vi "Chamber controller Dec 8 2016.vi"() -> ()   [LabVIEW 2014]
uses:
  <vilib>/Instr/_visa.llb/VISA Configure Serial Port (Instr).vi
  Environmental Chamber LabVIEW and Instruments/Drivers and Software/Keithley 2100 Series/Public/Configure/Configure 2 Wire Resistance.vi
  <vilib>/Utility/file.llb/Write To Spreadsheet File (string).vi
  <vilib>/Utility/file.llb/Read From Spreadsheet File (string).vi
  Environmental Chamber LabVIEW and Instruments/Drivers and Software/keithley_6430/Keithley 6430/Public/Data/Read (Single Point).vi
  Environmental Chamber LabVIEW and Instruments/Drivers and Software/LabVIEW 8.2 Drivers/keithley_24xx/Keithley 24XX/Public/Data/Read (Single Point).vi
  Environmental Chamber LabVIEW and Instruments/Drivers and Software/keithley_24xx/Keithley 24XX/Keithley 24XX.lvlib
  Environmental Chamber LabVIEW and Instruments/Drivers and Software/keithley_6430/Keithley 6430/Keithley 6430.lvlib
  Environmental Chamber LabVIEW and Instruments/Drivers and Software/Keithley 2100 Series/Keithley 2100 Series.lvlib
panel:
  out "pressure chart":cluster{"pressure":dbl}(graph)
  out "arduino qcm stack plot":T1(graph)
  in  "K-2420 tab control":enum32{"K-2420 Measure", "K-2420 Apply bias"}(tab)
  out "K-2420 2":cluster{"Resistance":sgl}(graph)
  in  "Applied Voltage (V)":dbl min=-5.0 max=5.0 step=5e-06
  out "K-2420 4":cluster{"Applied Voltage (V)":dbl}(graph)
  out "saving data?":bool
  in  "Data logging settings":T2={"Save during sequence only"=TRUE, "Save now"=FALSE, "sec between data points"=0.0, "Current data file path"=path "", "Save sample names"={"QCM1"="", "QCM2"="", "QCM3"="", "QCM4"="", "QCM5"="", "QCM6"="", "SRS"="", "K-2420"="", "K-6430"="", "K-2100"=""}, "Experiment Notes"="", "Cluster"={"Gas:"="CO2", "Vapor:"="H2O"}} {"sec between data points" min=0.0 max=30.0 format="%#_13g"}
  in  "Sequence cluster":T3={"Save sequence"=FALSE, "Clear sequence"=FALSE, "Import sequence file"=FALSE, "Tare elapsed time"=TRUE, "Run Sequence"=FALSE, "Stop program when sequence ends"=TRUE, "User-defined\nsequence"=[], "Sequence end time"="", "Sequence\npreview"=[], "Current\nstep"=0, "Display"=0} caption="Sequence settings" {"Display" items=["pressure", "gas flow", "vapor flow", "bias"]}
  in  "Pressure parameters cluster":T4={"valve % open"=100.0, "Desired pressure"=0.0, "Vapor sccm"=0.0, "Gas sccm"=0.0, "Valve mode"=enum."% Open", "Pressure Mode"=enum."Abs. pressure", "analyte partial pressure"=23.8, "Turbo pump\nauto on"=TRUE, "Valve position (%)"=0.0, "read pressure"=0.0, "read vapor flow"=0.0, "read gas flow"=0.0} caption="Pressure settings" {"read gas flow" format="%#_3g"; "read vapor flow" format="%#_3g"; "read pressure" format="%#_7f"; "Valve position (%)" format="%#_3g"; "analyte partial pressure" min=0.0 max=100.0 step=5.0; "Gas sccm" min=0 max=200 step=5; "Vapor sccm" min=0 max=200 step=5; "Desired pressure" min=0.0 max=760.0 step=5.0; "valve % open" min=0.0 max=100.0 step=5.0 format="%#_2f"}
  out "J-KEM temp chart":dbl(graph)
  out "Elapsed time (min)":dbl
  out "State date/time":string caption="Start time"
  out "K-2100 (Ohm)":cluster{"Measurement":dbl}(graph) caption="K-2100"
  out "K-6430":cluster{"Measurement":dbl}(graph)
  in  "Gate time (s)":enum16{"0.1", "1.0 ", "10"}(ring)=enum."1.0 "
  out "Hz":dbl format="%#.7f"
  out "QCM plot":T5(graph)
  in  "Stop":bool
  in  "Clear all charts":bool
  out "ArduinoQCM cluster":T6 caption="Arduino QCM" {"6" format="%_8g"; "5" format="%_8g"; "4" format="%_8g"; "3" format="%_8g"; "2" format="%_8g"; "1" format="%#_10g"}
  out "O2 sensor output":dbl[](array[numeric]) caption="atm\nTorr"
  in  "rapidox O2 Sensor":bool
  in  "setnag O2 Pump":bool
  in  "Baud Rate 2":i32(ring)=2 items=["2400", "4800", "9600", "19200", "38400", "57600", "115200"]
  in  "Com Port":i32(ring) items=["Com 1", "Com 2", "Com 3", "Com 4", "Com 5", "Com 6", "COM 7", "COM 8", "COM 9", "COM 10", "COM 11", "COM 12", "com 13", "COM 14"]
  in  "Com Port 2":i32(ring) items=["Com 1", "Com 2", "Com 3", "Com 4", "Com 5", "Com 6", "COM 7", "COM 8", "COM 9", "COM 10", "COM 11", "COM 12", "com 13", "COM 14"]
  out "Waveform Chart":cluster{dbl}(graph)
  out "O2 Concentration (PPM)":dbl
  out "Waveform Chart 6":cluster{dbl}(graph)
  # "Currently Unused"
  # "SRS"
  # "100%"
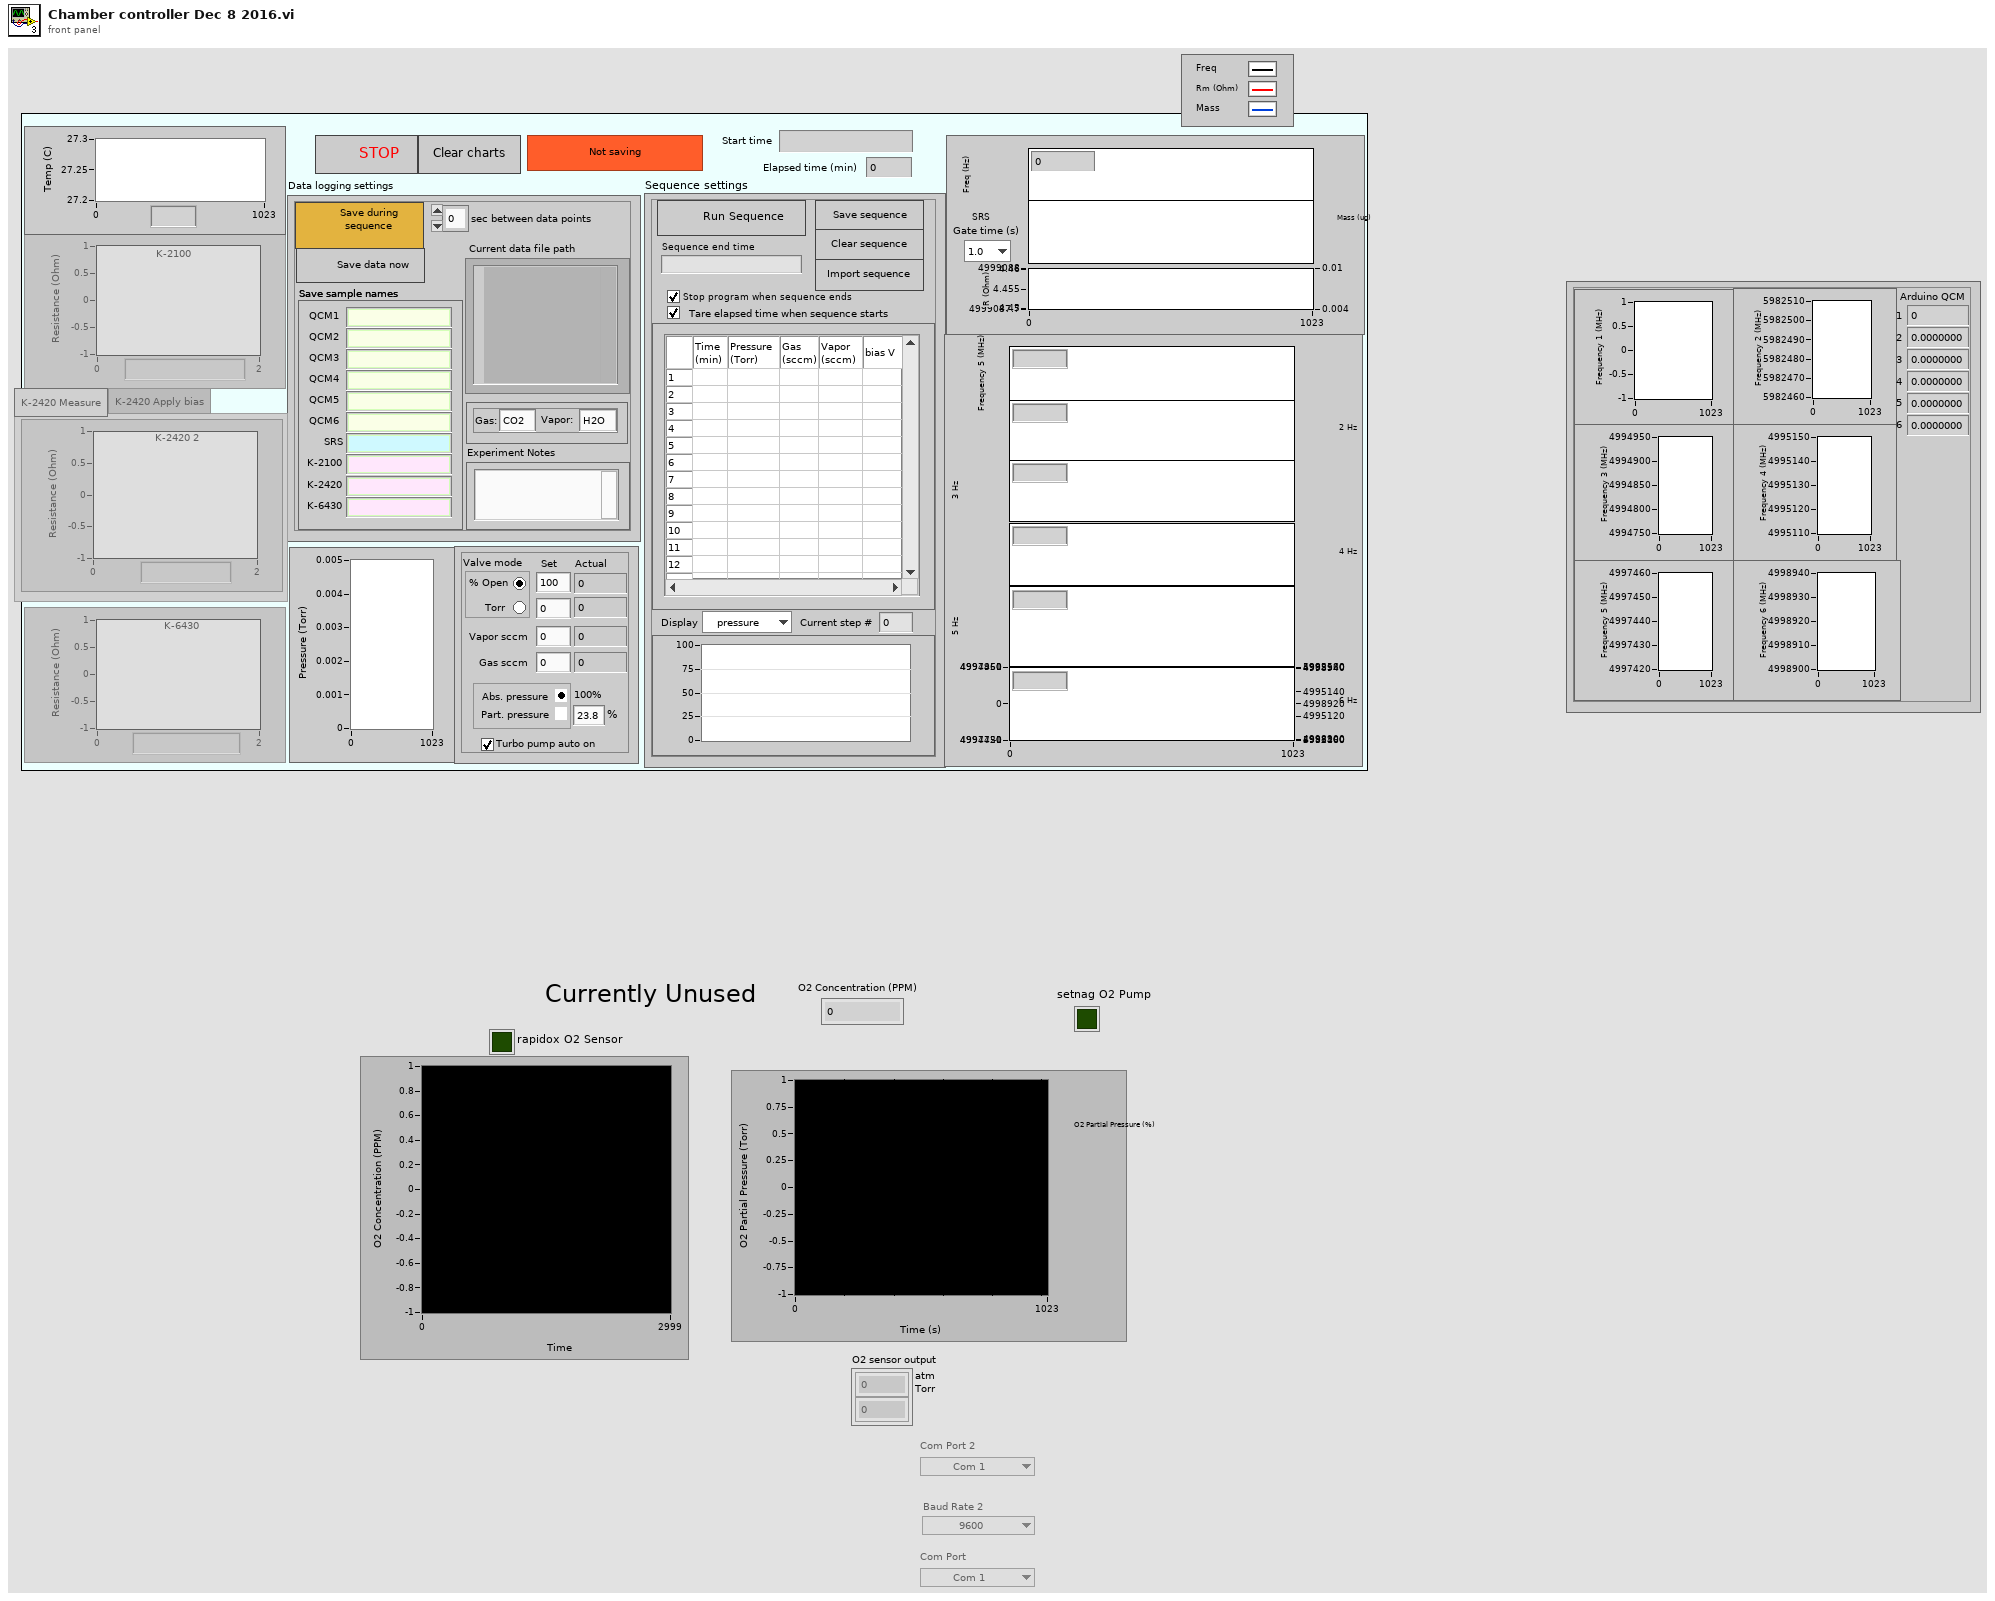
[diagram p1: front panel]
types:
  T1 = cluster{"mean":dbl, "mean":dbl, "mean":dbl, "mean":dbl, "mean":dbl, "mean":dbl}
  T2 = cluster{"Save during sequence only":bool, "Save now":bool, "sec between data points":dbl, "Current data file path":path, "Save sample names":cluster{"QCM1":string, "QCM2":string, "QCM3":string, "QCM4":string, "QCM5":string, "QCM6":string, "SRS":string, "K-2420":string, "K-6430":string, "K-2100":string}, "Experiment Notes":string, "Cluster":cluster{"Gas:":string, "Vapor:":string}}
  T3 = cluster{"Save sequence":bool, "Clear sequence":bool, "Import sequence file":bool, "Tare elapsed time":bool, "Run Sequence":bool, "Stop program when sequence ends":bool, "User-defined\nsequence":string[][], "Sequence end time":string, "Sequence\npreview":cluster{dbl[], dbl[]}[], "Current\nstep":i32, "Display":u16}
  T4 = cluster{"valve % open":dbl, "Desired pressure":dbl, "Vapor sccm":sgl, "Gas sccm":sgl, "Valve mode":enum32{"% Open", "Torr "}, "Pressure Mode":enum32{"Abs. pressure", " Part. pressure"}, "analyte partial pressure":dbl, "Turbo pump\nauto on":bool, "Valve position (%)":dbl, "read pressure":dbl, "read vapor flow":dbl, "read gas flow":dbl}
  T5 = cluster{"Frequency out":dbl, "Numeric Control":dbl, "Resistance out":dbl}
  T6 = cluster{"arduino qcm 1":dbl, "1":dbl, "arduino qcm 2":dbl, "2":dbl, "arduino qcm 3":dbl, "3":dbl, "arduino qcm 4":dbl, "4":dbl, "arduino qcm 5":dbl, "5":dbl, "arduino qcm 6":dbl, "6":dbl}
  T7 = cluster{"Keithley 6430":bool, "J-KEM":bool, "Keithley 2420":bool, "Keithley 2100":bool, "SRS QCM":bool, "Pressure control":bool, "Arduino":bool}
  T8 = cluster{"Arduino 1":refnum<visa-resource-name>, "Arduino 2":refnum<visa-resource-name>, "Arduino 3":refnum<visa-resource-name>, "Arduino 4":refnum<visa-resource-name>, "Arduino 5":refnum<visa-resource-name>, "Arduino 6":refnum<visa-resource-name>}
  T9 = enum8{"Enabled", "Disabled", "Disabled and Grayed Out"}
  T10 = enum16{"open", "open or create", "create or replace", "create", "open (read only)"}
  T11 = enum16{"no parity", "odd parity", "even parity", "mark parity", "space parity"}
  T12 = cluster{"mean":dbl, "mean":dbl, "mean":dbl, "mean":dbl, "mean":dbl, "mean":dbl}[]
  T13 = cluster{"Frequency out":dbl, "Numeric Control":dbl, "Resistance out":dbl}[]
  T14 = cluster{"String":string, "String":string, "String":string}
  T15 = cluster{bool, "task out":refnum<k21>, "error out":errorcluster, "task out":refnum<k21>, "error out":errorcluster, "turbo pump":refnum<visa-resource-name>, "error out":errorcluster}
  T16 = cluster{bool, "task out":refnum<k21>, "error out":errorcluster, "task out":refnum<k21>, "error out":errorcluster, "VISA resource name out":refnum<visa-resource-name>, "error out":errorcluster}
  T17 = cluster{bool, "VISA resource name":refnum<visa-resource-name>, "error out":errorcluster}
  T18 = cluster{bool, "VISA resource name out":refnum<visa-resource-name>, "error out":errorcluster}
  T19 = cluster{"VISA resource name out":refnum<visa-resource-name>, "error out":errorcluster, "VISA resource name out":refnum<visa-resource-name>, "error out":errorcluster, "VISA resource name out":refnum<visa-resource-name>, "error out":errorcluster, "VISA resource name out":refnum<visa-resource-name>, "error out":errorcluster, "VISA resource name out":refnum<visa-resource-name>, "error out":errorcluster, "VISA resource name out 2":refnum<visa-resource-name>, "error out 2":errorcluster}
  T20 = cluster{"Boolean":bool, "VISA resource name out":refnum<visa-resource-name>, "error out":errorcluster}
  T21 = cluster{bool, "VISA out":refnum<visa-resource-name>, "error out":errorcluster}
  T22 = cluster{"Boolean":bool, "VISA out":refnum<visa-resource-name>, "error out":errorcluster}
  T23 = cluster{"Numeric Control":dbl, "Cluster":cluster{"Numeric Control":dbl}, "String":string, "error out":errorcluster}
  T24 = cluster{bool, "Com Port":i32, "Numeric Control out":dbl}
  T25 = cluster{"Arduino address":refnum<visa-resource-name>, "error in (no error)":errorcluster, "Arduino address 2":refnum<visa-resource-name>, "error in (no error) 2":errorcluster, "Arduino address 3":refnum<visa-resource-name>, "error in (no error) 3":errorcluster, "Arduino address 4":refnum<visa-resource-name>, "error in (no error) 4":errorcluster, "Arduino address 5":refnum<visa-resource-name>, "error in (no error) 5":errorcluster, "Arduino address 6":refnum<visa-resource-name>, "error in (no error) 6":errorcluster}
  T26 = cluster{"mean":string, "mean":string, "mean":string, "mean":string, "mean":string, "mean":string}
  T27 = cluster{"valve % open":dbl, "Desired pressure":dbl, "Vapor sccm":sgl, "Gas sccm":sgl, "Valve mode":enum32{"% Open", "Torr "}, "Pressure Mode":enum32{"Abs. pressure", " Part. pressure"}, "analyte partial pressure":dbl}
  T28 = cluster{"User-defined\nsequence":string[][], "Present (s)":dbl, "current  step # in":i32, "sequence end time in":timestamp}
  T29 = cluster{"current  step # in":i32, "sequence end time in":timestamp, "Boolean":bool}
  T30 = cluster{"press/RH/gas/vapor":cluster{"pressure":string, "RH":string, "gas flow":string, "vapor flow":string}, "Cluster":cluster{"Valve position (%)":dbl, "read pressure":dbl, "read vapor flow":dbl, "read gas flow":dbl}}
  T31 = cluster{"Boolean":bool, "task out":refnum<k21>, "error out":errorcluster, "task out":refnum<k21>, "error out":errorcluster, "VISA resource name out":refnum<visa-resource-name>, "error out":errorcluster}
  T32 = cluster{"pressure":string, "RH":string, "gas flow":string, "vapor flow":string}
  T33 = cluster{"Valve position (%)":dbl, "read pressure":dbl, "read vapor flow":dbl, "read gas flow":dbl}
  T34 = cluster{"f":dbl, "f":dbl, "f":dbl, "f":dbl, "f":dbl}[]
  T35 = cluster{"QCM1":string, "QCM2":string, "QCM3":string, "QCM4":string, "QCM5":string, "QCM6":string, "SRS":string, "K-2420":string, "K-6430":string, "K-2100":string}
  T36 = cluster{"mean":dbl, "mean":dbl, "mean":dbl, "mean":dbl, "mean":dbl, "mean":dbl, "mean":dbl, "mean":dbl, "mean":dbl, "mean":dbl, "mean":dbl, "mean":dbl}
  T37 = cluster{"String data out":string, string, string, string}
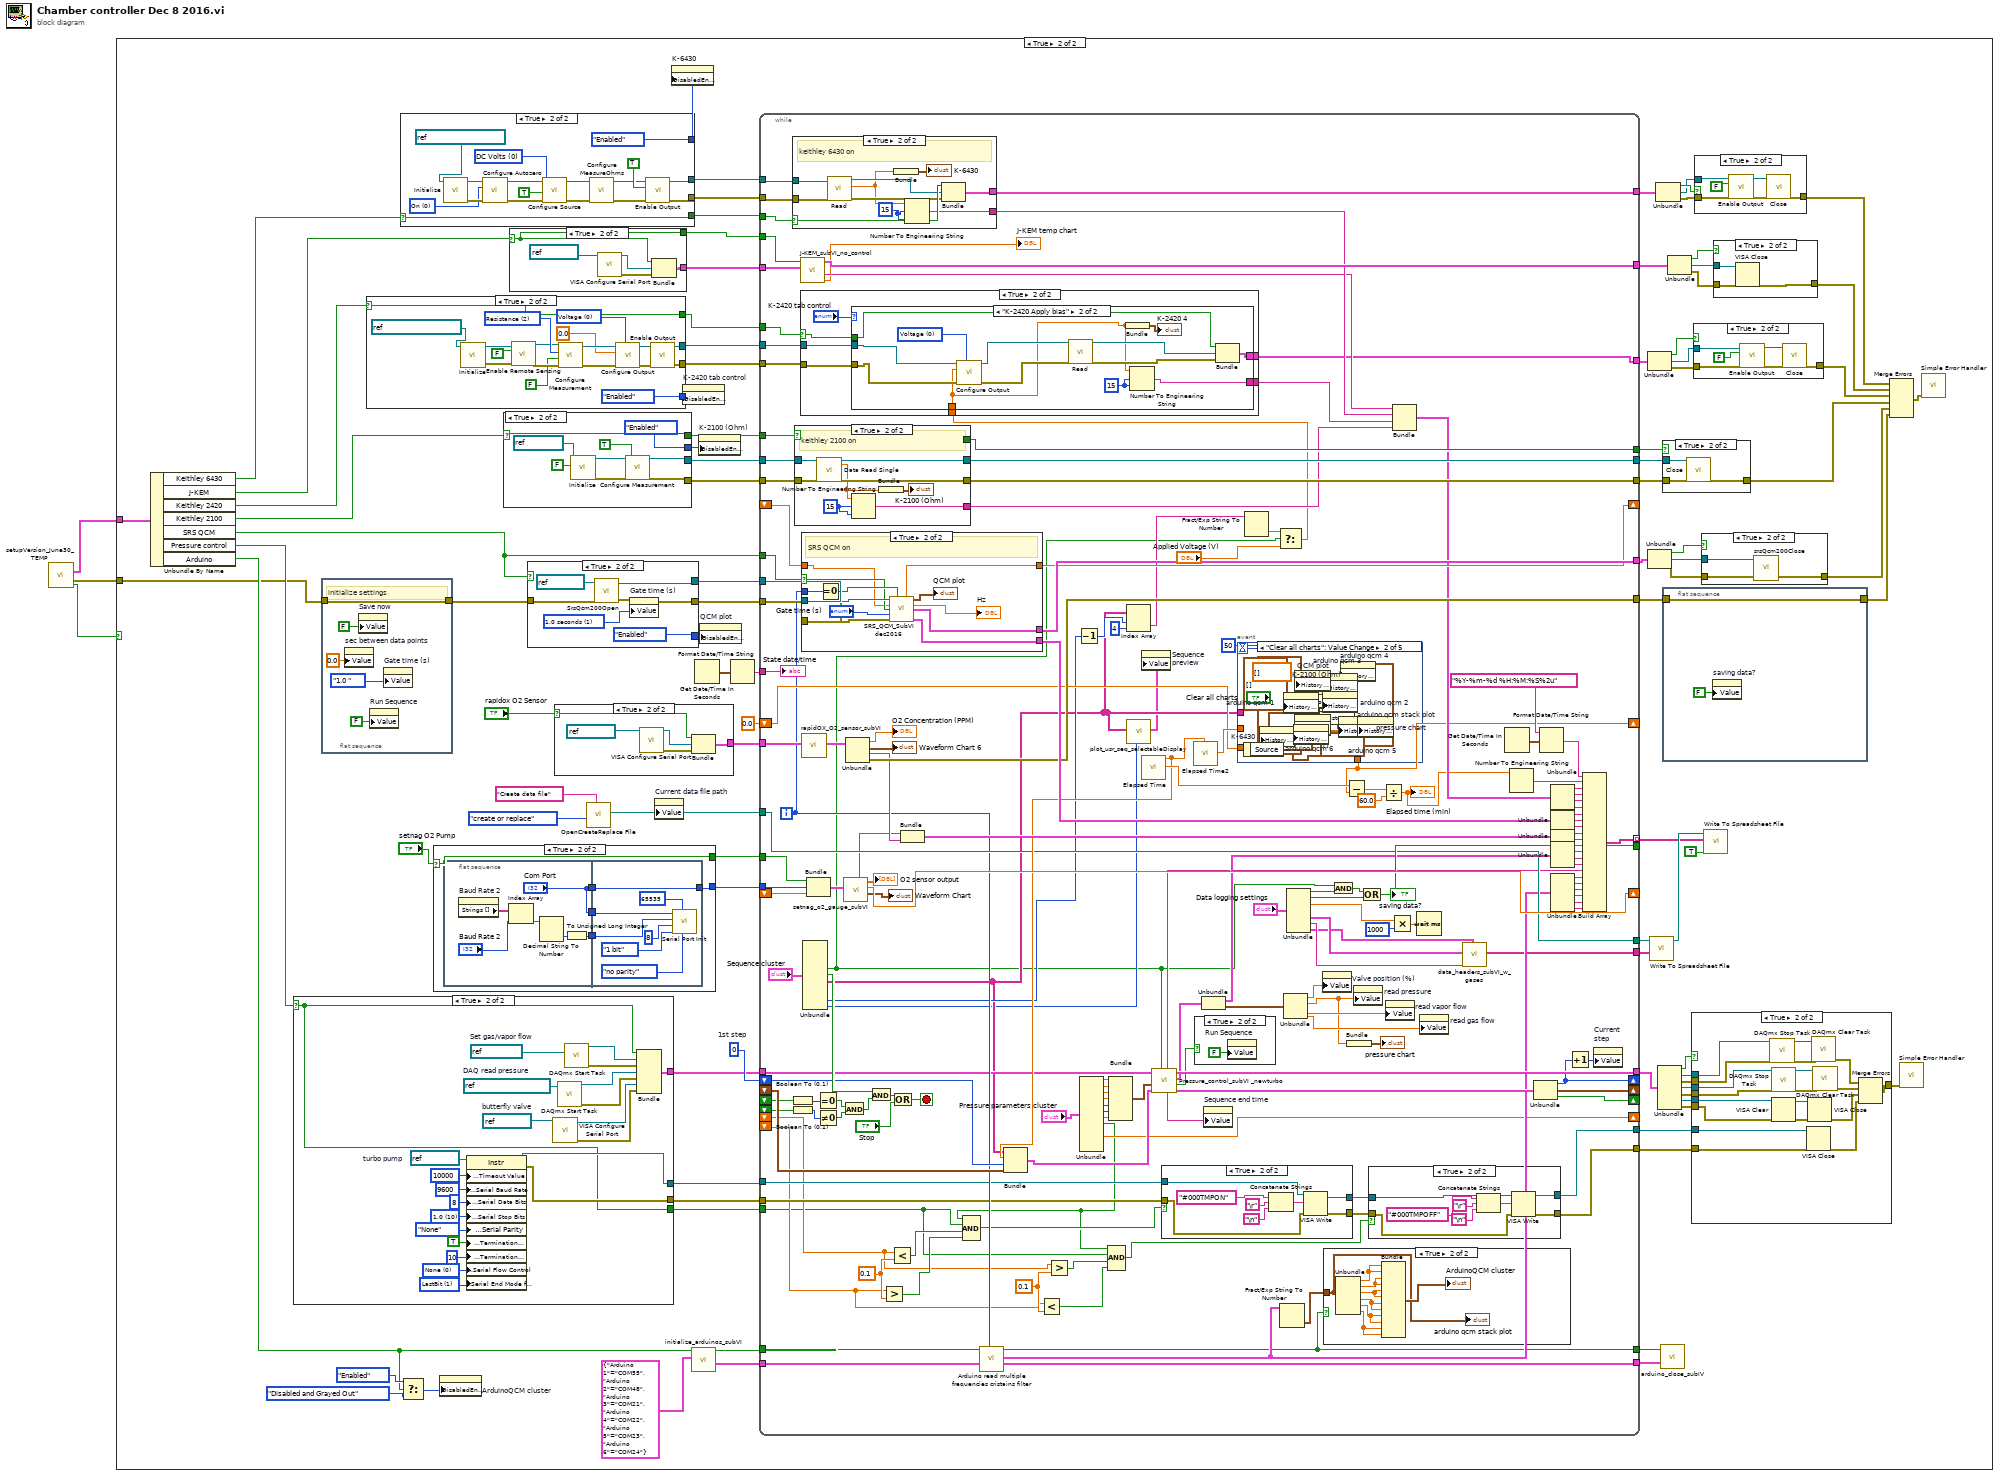
[diagram p0: block diagram]
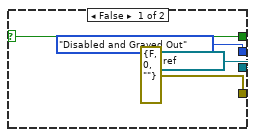
[diagram p4: hidden frame]
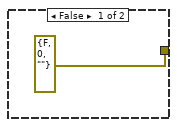
[diagram p5: hidden frame]
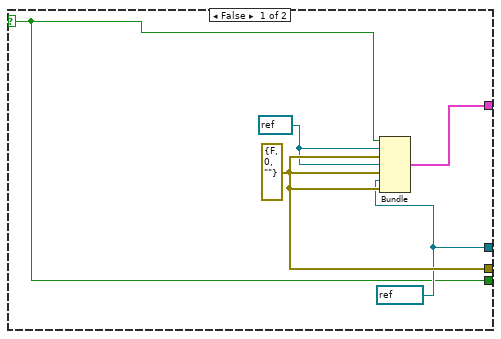
[diagram p6: hidden frame]
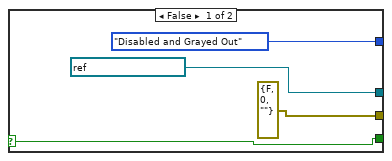
[diagram p8: hidden frame]
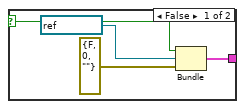
[diagram p9: hidden frame]
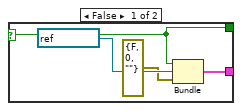
[diagram p11: hidden frame]
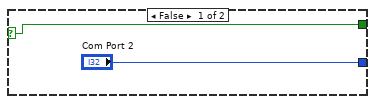
[diagram p12: hidden frame]
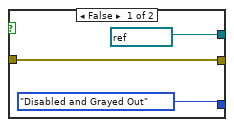
[diagram p14: hidden frame]
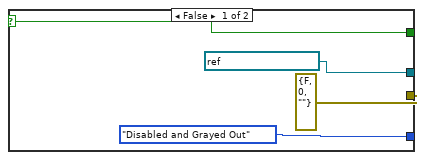
[diagram p16: hidden frame]
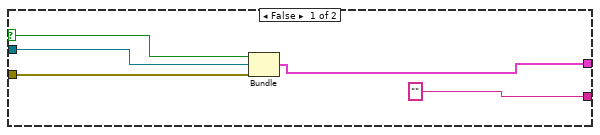
[diagram p17: hidden frame]
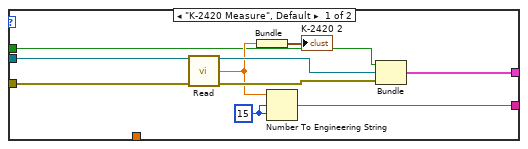
[diagram p18: hidden frame]
diagram:
  n1 = call "setupVersion_June30_TEMP.vi"() -> ("Instruments on/off"=w1:T7, "error IO"=w2:errorcluster, "OK"=w3:bool)  [unwired: 13 in]
  n2 = case shown="True" w3 {
    tunnel: w2 -> [_ w19]
    tunnel: w1 -> [_ w29]
    frame False {
    }
    frame True {
      w35 = 0  # 1st step
      n3 = Unbundle By Name(w29) -> ("Keithley 6430"=w28:bool, "J-KEM"=w27:bool, "Keithley 2420"=w26:bool, "Keithley 2100"=w25:bool, "SRS QCM"=w24:bool, "Pressure control"=w23:bool, "Arduino"=w22:bool)
      n4 = case shown="True" w23 {
        selector: w23 -> [w142 w147]
        tunnel: [w146 w148] -> w17
        tunnel: [w145 w150] -> w9
        tunnel: [w143 w149] -> w10
        tunnel: [w142 w147] -> w8
        frame False {
          w143 = refnum<visa-resource-name> refnum ("turbo pump")
          w144 = refnum<k21> refnum ("task out")
          w145 = errorcluster {"status"=FALSE, "code"=0, "source"=""} ("error out")
          n5 = Bundle(w142, "task out"=w144, "error out"=w145, "task out"=w144, "error out"=w145, "turbo pump"=w143, "error out"=w145) -> (w146:T15)  [unwired: 1 in]
        }
        frame True {
          w154 = u16 1 items=["None", "LastBit", "TermChar"] ("Serial Settings:Serial End Mode for Reads")
          w152 = u16 0 items=["None", "XON/XOFF", "RTS/CTS", "XON/XOFF & RTS/CTS", "DTR/DSR", "XON/XOFF & DTR/DSR"] ("flow control (0:none)")
          w155 = u16 10 items=["1.0"=10, "1.5"=15, "2.0"=20] ("stop bits (10: 1 bit)")
          w151 = refnum<visa-resource-name> "COM7"  # turbo pump
          w167 = refnum<visa-resource-name> "COM5"  # butterfly valve
          w168 = refnum<k21> "Setflow"  # Set gas/vapor flow
          w169 = refnum<k21> "AllDaqReadings"  # DAQ read pressure
          n6 = property class="Instr"(reference=w151, "General Settings:Timeout Value"=u32 10000 ("timeout (10sec)"), "Serial Settings:Serial Baud Rate"=u32 9600 ("baud rate (9600)"), "Serial Settings:Serial Data Bits"=u16 8 ("data bits (8)"), "Serial Settings:Serial Stop Bits"=w155, "Serial Settings:Serial Parity"=enum16{"None", "Odd", "Even", "Mark", "Space"}."None" ("parity (0:none)"), "Message Based Settings:Termination Character Enable"=TRUE ("Enable Termination\nChar (T)"), "Message Based Settings:Termination Character"=u8 10 ("termination char\n(0xA = '\\n' = LF)"), "Serial Settings:Serial Flow Control"=w152, "Serial Settings:Serial End Mode for Reads"=w154) -> (reference out=w149:refnum<visa-resource-name>, error out=w150:errorcluster)  [unwired: 1 in]
          n7 = call-poly "VISA Configure Serial Port"("VISA resource name"=w167) -> ("VISA resource name out"=w162:refnum<visa-resource-name>, "error out"=w161:errorcluster)  [unwired: 13 in]
          n8 = call <vilib>:"DAQmx Start Task.vi"("task/channels in"=w169) -> ("task out"=w164:refnum<k21>, "error out"=w163:errorcluster)  [unwired: 13 in]
          n9 = call <vilib>:"DAQmx Start Task.vi"("task/channels in"=w168) -> ("task out"=w166:refnum<k21>, "error out"=w165:errorcluster)  [unwired: 13 in]
          n10 = Bundle(w147, "task out"=w166, "error out"=w165, "task out"=w164, "error out"=w163, "VISA resource name out"=w162, "error out"=w161) -> (w148:T16)  [unwired: 1 in]
        }
      }
      n11 = flat-sequence {
        tunnel: [w98] -> w18
        tunnel: w19 -> [w98]
        frame #0 {
          # "initialize settings"
          n12 = property on="sec between data points" class="DigNum (strict)"("Value"=0.0) -> ()  [unwired: 2 in, 2 out]
          n13 = property on="Save now" class="Bool (strict)"("Value"=FALSE) -> ()  [unwired: 2 in, 2 out]
          n14 = property on="Run Sequence" class="Bool (strict)"("Value"=FALSE) -> ()  [unwired: 2 in, 2 out]
          n15 = property on="Gate time (s)" class="Enum (strict)"("Value"=enum16{"0.1", "1.0 ", "10"}."1.0 " ("Gate time (sec)")) -> ()  [unwired: 2 in, 2 out]
        }
      }
      n16 = case shown="True" w26 {
        selector: w26 -> [w261 w265]
        tunnel: [refnum<visa-resource-name> "GPIB1::24::INSTR" ("VISA resource name") w274] -> w95
        tunnel: [errorcluster {"status"=FALSE, "code"=0, "source"=""} ("error out") w269] -> w94
        tunnel: [T9."Disabled and Grayed Out" ("Disabled") T9."Enabled" ("Disabled")] -> w58
        tunnel: [w261 w265] -> w51
        frame False {
        }
        frame True {
          w276 = u16 0 items=["Voltage", "Current"] ("Source Mode  (0: Voltage)")
          w281 = u16 2 items=["Volts", "Current", "Resistance"] ("Function (0: Volts)")
          n17 = call "Initialize.vi"("VISA resource name"=refnum<visa-resource-name> "GPIB1::24::INSTR") -> ("error out"=w270:errorcluster, "VISA resource name out"=w273:refnum<visa-resource-name>)  [unwired: 9 in]
          n18 = call "Enable Remote Sensing.vi"("error in (no error)"=w270, "Enable Remote Sensing (T: Enable)"=FALSE ("4-wire?"), "VISA resource name"=w273) -> ("error out"=w271:errorcluster, "VISA resource name out"=w272:refnum<visa-resource-name>)  [unwired: 7 in]
          n19 = call "Configure Measurement.vi"("error in (no error)"=w271, "Enable Auto Range (T:Enable)"=FALSE, "Function (0: Volts)"=w281, "VISA resource name"=w272) -> ("error out"=w280:errorcluster, "VISA resource name out"=w279:refnum<visa-resource-name>)  [unwired: 6 in]
          n20 = call "Configure Output.vi"("Source Mode  (0: Voltage)"=w276, "error in (no error)"=w280, "Output Level (0)"=0.0 ("Applied Voltage (V)"), "VISA resource name"=w279) -> ("error out"=w278:errorcluster, "VISA resource name out"=w277:refnum<visa-resource-name>)  [unwired: 6 in]
          n21 = call "Enable Output.vi"("error in (no error)"=w278, "VISA resource name"=w277) -> ("error out"=w269:errorcluster, "VISA resource name out"=w274:refnum<visa-resource-name>)  [unwired: 8 in]
        }
      }
      n22 = case shown="True" w28 {
        selector: w28 -> [w177 w181]
        tunnel: [refnum<visa-resource-name> "GPIB0::29::INSTR" ("VISA resource name") w192] -> w64
        tunnel: [errorcluster {"status"=FALSE, "code"=0, "source"=""} ("error out") w193] -> w63
        tunnel: [T9."Disabled and Grayed Out" ("Disabled") T9."Enabled" ("Disabled")] -> w57
        tunnel: [w177 w181] -> w50
        frame False {
        }
        frame True {
          w182 = u16 0 items=["DC Volts", "DC Current"] ("Source Function (0: DC Volts)")
          w189 = u16 0 items=["On", "Off", "Once"] ("Autozero  (0: On)")
          n23 = call "Initialize.vi"("VISA resource name"=refnum<visa-resource-name> "GPIB0::29::INSTR") -> ("error out"=w190:errorcluster, "VISA resource name out"=w191:refnum<visa-resource-name>)  [unwired: 4 in, 5 out]
          n24 = call "Configure Autozero.vi"("error in (no error)"=w190, "Autozero  (0: On)"=w189, "VISA resource name"=w191) -> ("error out"=w185:errorcluster, "VISA resource name out"=w187:refnum<visa-resource-name>)  [unwired: 7 in]
          n25 = call "Configure Source.vi"("error in (no error)"=w185, "Auto Range (T:Enable)"=TRUE, "Source Function (0: DC Volts)"=w182, "VISA resource name"=w187) -> ("error out"=w184:errorcluster, "VISA resource name out"=w186:refnum<visa-resource-name>)  [unwired: 6 in]
          n26 = call "Configure MeasureOhms.vi"("error in (no error)"=w184, "VISA resource name"=w186) -> ("error out"=w197:errorcluster, "VISA resource name out"=w195:refnum<visa-resource-name>)  [unwired: 4 in, 4 out]
          n27 = call "Enable Output.vi"("error in (no error)"=w197, "Enable Output (F:Off)"=TRUE ("Output (F:Off)"), "VISA resource name"=w195) -> ("error out"=w193:errorcluster, "VISA resource name out"=w192:refnum<visa-resource-name>)  [unwired: 7 out]
        }
      }
      n28 = Select(t=T9."Enabled" ("Disabled"), s=w22, f=T9."Disabled and Grayed Out" ("Disabled")) -> (s? t:f=w4:T9)
      n29 = case shown="True" "setnag O2 Pump" {
        selector: "setnag O2 Pump" -> [w220 w222]
        tunnel: ["Com Port 2" w223] -> w91
        tunnel: [w220 w222] -> w40
        frame False {
        }
        frame True {
          n30 = flat-sequence {
            tunnel: ["Com Port"] -> w226
            tunnel: [w228] -> w225
            tunnel: ["Com Port"] -> w224
            tunnel: w226 -> [w234]
            tunnel: w225 -> [w233]
            tunnel: w224 -> [w235]
            tunnel: [w235] -> w223
            frame #0 {
              n31 = property on="Baud Rate 2" class="Ring (strict)"() -> ("Strings []"=w230:string[])  [unwired: 2 in, 2 out]
              n32 = Index Array(array=w230, index="Baud Rate 2") -> (element=w231:string)
              n33 = Decimal String To Number(string=w231) -> (number=w229:i32)  [unwired: 2 in, 1 out]
              n34 = To Unsigned Long Integer(number=w229) -> (unsigned 32bit integer=w228:u32)
            }
            frame #1 {
              n35 = call <vilib>:"Serial Port Init.vi"("parity"=T11."no parity", "buffer size"=u16 65535, "stop bits"=enum16{"1 bit", "1.5 bits", "2 bits"}."1 bit", "data bits"=u16 8, "baud rate"=w233, "port number"=w234) -> ()  [unwired: 1 in, 1 out]
            }
          }
        }
      }
      n36 = property on="ArduinoQCM cluster" class="Clust (strict)"("DisabledEnum"=w4) -> ()  [unwired: 2 in, 2 out]
      n37 = case shown="True" w25 {
        selector: w25 -> [w110 w115]
        tunnel: [refnum<visa-resource-name> "K-2100" ("VISA resource name out") w118] -> w49
        tunnel: [errorcluster {"status"=FALSE, "code"=0, "source"=""} ("error out") w117] -> w48
        tunnel: [w110 w115] -> w47
        tunnel: [T9."Disabled and Grayed Out" ("Disabled") T9."Enabled" ("Disabled")] -> w42
        frame False {
        }
        frame True {
          n38 = call "Initialize.vi"("VISA resource name"=refnum<visa-resource-name> "K-2100", "Reset? (T: Reset)"=FALSE) -> ("VISA resource name out"=w119:refnum<visa-resource-name>, "error out"=w116:errorcluster)  [unwired: 16 in]
          n39 = call-poly "Configure Measurement.vi"("VISA resource name"=w119, "error in (no error)"=w116, "Auto Range? (T: Auto)"=TRUE) -> ("VISA resource name out"=w118:refnum<visa-resource-name>, "error out"=w117:errorcluster)  [unwired: 15 in]
        }
      }
      n40 = case shown="True" w27 {
        selector: w27 -> [w211 w216]
        tunnel: [w212 w217] -> w80
        tunnel: [w211 w216] -> w74
        frame False {
          n41 = Bundle(w211, "VISA resource name"=refnum<visa-resource-name> "COM3", "error out"=errorcluster {"status"=FALSE, "code"=0, "source"=""}) -> (w212:T17)  [unwired: 1 in]
        }
        frame True {
          n42 = call-poly "VISA Configure Serial Port"("VISA resource name"=refnum<visa-resource-name> "COM3") -> ("VISA resource name out"=w218:refnum<visa-resource-name>, "error out"=w215:errorcluster)  [unwired: 13 in]
          n43 = Bundle(w216, "VISA resource name out"=w218, "error out"=w215) -> (w217:T18)  [unwired: 1 in]
        }
      }
      n44 = case shown="True" w24 {
        tunnel: [refnum<visa-resource-name> "COM6" ("VISA in") w250] -> w93
        tunnel: [w245 w247] -> w92
        tunnel: w18 -> [w245 w252]
        tunnel: [T9."Disabled and Grayed Out" ("Disabled") T9."Enabled" ("Disabled")] -> w59
        frame False {
        }
        frame True {
          w249 = u16 1 items=["0.1 seconds", "1.0 seconds", "10.0 seconds"] ("Gate time")
          n45 = call "SrsQcm200Open.vi"("error in"=w252, "VISA in"=refnum<visa-resource-name> "COM6") -> ("error out"=w248:errorcluster, "VISA out"=w250:refnum<visa-resource-name>)  [unwired: 3 in]
          n46 = property on="Gate time (s)" class="Enum (strict)"(error in=w248, "Value"=w249) -> (error out=w247:errorcluster)  [unwired: 1 in, 1 out]
        }
      }
      n47 = case shown="True" "rapidox O2 Sensor" {
        selector: "rapidox O2 Sensor" -> [w198 w203]
        tunnel: [w199 w204] -> w70
        frame False {
          n48 = Bundle(w198, "VISA resource name"=refnum<visa-resource-name> "COM7", "error out"=errorcluster {"status"=FALSE, "code"=0, "source"=""}) -> (w199:T17)  [unwired: 1 in]
        }
        frame True {
          n49 = call-poly "VISA Configure Serial Port"("VISA resource name"=refnum<visa-resource-name> "COM7") -> ("VISA resource name out"=w205:refnum<visa-resource-name>, "error out"=w202:errorcluster)  [unwired: 13 in]
          n50 = Bundle(w203, "VISA resource name out"=w205, "error out"=w202) -> (w204:T18)  [unwired: 1 in]
        }
      }
      n51 = call "OpenCreateReplace File.vi"("prompt"="Create data file", "function (open:0)"=T10."create or replace") -> ("new file path"=w5:path)  [unwired: 6 in, 3 out]
      n52 = property on="Current data file path" class="Path"("Value"=w5) -> ()  [unwired: 2 in, 2 out]
      n53 = property on="K-6430" class="WFChart (strict)"("DisabledEnum"=w57) -> ()  [unwired: 2 in, 2 out]
      n54 = property on="K-2420 tab control" class="TabCtl (strict)"("DisabledEnum"=w58) -> ()  [unwired: 2 in, 2 out]
      n55 = call "initialize_arduinos_subVI.vi"("arduino 1-6 addresses"=T8 {"Arduino 1"="COM55", "Arduino 2"="COM48", "Arduino 3"="COM21", "Arduino 4"="COM22", "Arduino 5"="COM23", "Arduino 6"="COM24"} ("Arduino COMs"), "arduinos on?"=w22) -> ("arduino addresses/errors"=w36:T19, "arduinos on/off"=w55:bool)  [unwired: 8 in]
      n56 = Get Date/Time In Seconds() -> (seconds since 1Jan1904=w97:timestamp)
      n57 = property on="K-2100 (Ohm)" class="WFChart (strict)"("DisabledEnum"=w42) -> ()  [unwired: 2 in, 2 out]
      n58 = property on="QCM plot" class="WFChart (strict)"("DisabledEnum"=w59) -> ()  [unwired: 2 in, 2 out]
      n59 = Format Date/Time String(seconds (now)=w97) -> (date/time string=w39:string)  [unwired: 2 in]
      n60 = while {
        shift-right: [w452] -> _
        shift-left: _ -> [w389]
        tunnel: [w440] -> w56 mode=indexing if=w410
        tunnel: w51 -> [w291]
        tunnel: w95 -> [w293]
        tunnel: w94 -> [w292]
        tunnel: w93 -> [w451]
        tunnel: w92 -> [w450]
        tunnel: w24 -> [w449]
        tunnel: w40 -> [w391]
        tunnel: w91 -> [w392]
        tunnel: [w285] -> w88
        tunnel: [w448] -> w84
        tunnel: w80 -> [w447]
        tunnel: [w446] -> w79
        tunnel: w74 -> [w445]
        tunnel: w70 -> [w399]
        tunnel: [w395] -> w21
        tunnel: [w338] -> w69
        tunnel: w5 -> [w338]
        shift-right: [w438] -> _
        shift-left: _ -> [w439]
        tunnel: w64 -> [w444]
        tunnel: w63 -> [w443]
        tunnel: [w442] -> w62
        tunnel: [w410] -> _
        tunnel: w55 -> [w327]
        tunnel: w36 -> [w330]
        tunnel: [w326] -> w53
        tunnel: [w328] -> w54
        tunnel: [w296] -> w52
        tunnel: w50 -> [w422]
        tunnel: w49 -> [w409]
        tunnel: w48 -> [w408]
        tunnel: w47 -> [w407]
        tunnel: [w406] -> w46
        tunnel: [w405] -> w45
        tunnel: [w404] -> w44
        shift-right: [w383] -> _
        shift-left: 0.0 ("Elapsed Time (s)") -> [w384]
        tunnel: w39 -> [w374]
        tunnel: w17 -> [w323]
        shift-right: [w335] -> _
        shift-left: w35 -> [w349]
        shift-right: [w355] -> _
        shift-left: _ -> [w353]
        shift-right: [w354] -> _
        shift-left: _ -> [w352]
        shift-left: _ -> [w351]
        tunnel: [w347] -> w34
        tunnel: w10 -> [w318]
        tunnel: w9 -> [w317]
        tunnel: w8 -> [w307]
        tunnel: [w312] -> w7
        tunnel: [w313] -> w6
        shift-right: [w322] -> _
        shift-left: _ -> [w309]
        shift-left: _ -> [w308]
        i -> [w325]
        stop <- w412 stop-if-true
        w311 = 0.1 ("y")
        w321 = 0.1 ("y")
        n61 = Boolean To (0,1)(Boolean=w352) -> (0, 1=w420:i16)
        n62 = Boolean To (0,1)(Boolean=w351) -> (0, 1=w419:i16)
        n63 = case "Keithley 6430" shown="True" w422 {
          selector: w422 -> [w543 w554]
          tunnel: w444 -> [w542 w551]
          tunnel: w443 -> [w541 w550]
          tunnel: ["" w553] -> w394
          tunnel: [w540 w552] -> w442
          frame False {
            # "keithley 6430 off"
            n64 = Bundle(w543, "VISA resource name out"=w542, "error out"=w541) -> (w540:T18)  [unwired: 1 in]
          }
          frame True {
            w545 = i16 15 ("width (-)")
            # "keithley 6430 on"
            n65 = call-poly "Read.vi"("error in (no error)"=w550, "VISA resource name"=w551) -> ("error out"=w549:errorcluster, "Measurement"=w547:dbl, "VISA resource name out"=w548:refnum<visa-resource-name>)  [unwired: 1 in, 6 out]
            n66 = Bundle("Measurement"=w547) -> (→"K-6430":cluster{"Measurement":dbl})  [unwired: 1 in]
            n67 = Number To Engineering String(2:w545, 3:w545, 4:w547) -> (0:w553:string)  [unwired: 1 in]
            n68 = Bundle(w554, "VISA resource name out"=w548, "error out"=w549) -> (w552:T18)  [unwired: 1 in]
          }
        }
        n69 = case shown="True" w407 {
          selector: w407 -> [w518 w523]
          tunnel: [w519 w530] -> w405
          tunnel: [w520 w529] -> w404
          tunnel: w409 -> [w519 w528]
          tunnel: w408 -> [w520 w527]
          tunnel: ["" w525] -> w393
          tunnel: [w518 w523] -> w406
          frame False {
            # "keithley 2100 off"
          }
          frame True {
            w522 = i16 15 ("width (-)")
            # "keithley 2100 on"
            n70 = call "Data Read Single.vi"("VISA resource name"=w528, "error in (no error)"=w527) -> ("VISA resource name out"=w530:refnum<visa-resource-name>, "Measurement"=w526:dbl, "error out"=w529:errorcluster)  [unwired: 15 in]
            n71 = Number To Engineering String ("elapsed time (min)")(2:w522, 3:w522, 4:w526) -> (0:w525:string)  [unwired: 1 in]
            n72 = Bundle("Measurement"=w526) -> (→"K-2100 (Ohm)":cluster{"Measurement":dbl})  [unwired: 1 in]
          }
        }
        n73 = call "J-KEM_subVI_no_control.vi"("Address in"=w447, "J-KEM on?"=w445) -> ("Temp (C)"=→"J-KEM temp chart":dbl, "String data out"=w382:string, "Address out"=w446:T20)  [unwired: 6 in, 1 out]
        n74 = case "SRS QCM" shown="True" w449 {
          selector: w449 -> [w557 w567]
          tunnel: w451 -> [w560 w569]
          tunnel: w450 -> [w559 w571]
          tunnel: [w558 w564] -> w448
          tunnel: w439 -> [w555 w565]
          tunnel: [w555 w566] -> w438
          tunnel: [T14 {"String"="", "String"="", "String"=""} ("M,F,MR output cluster") w563] -> w431
          tunnel: w325 -> [_ w572]
          frame False {
            # "SRS QCM off"
            n75 = Bundle(w557, "VISA out"=w560, "error out"=w559) -> (w558:T21)  [unwired: 1 in]
          }
          frame True {
            # "SRS QCM on"
            n76 = Equal To 0?(x=w572) -> (x = 0?=w568:bool)
            n77 = call "SRS_QCM_SubVI  dec2016.vi"("VISA Refnum in"=w569, "first iteration?"=w568, "Frequency  in"=w565, "SRS on?"=w567, "Gate time"="Gate time (s)", "error in (no error)"=w571) -> ("Frequency out 2"=w566:dbl, "freq, mass, MR"=→"QCM plot":T5, "Frequency out"=→"Hz":dbl, "address out"=w564:T22, "M,F,MR output cluster"=w563:T14)  [unwired: 2 in, 3 out]
          }
        }
        n78 = call "rapidOX_O2_sensor_subVI.vi"("rapid ox info in"=w399) -> ("rapidox info out"=w398:T23)  [unwired: 10 in]
        n79 = Unbundle("Sequence cluster") -> ("Run Sequence"=w286:bool, "Stop program when sequence ends"=w350:bool, "User-defined\nsequence"=w300:string[][], "Current\nstep"=w302:i32, "Display"=w298:u16)  [unwired: 6 out]
        n80 = Bundle(w391, "Com Port"=w392, "Numeric Control out"=w389) -> (w390:T24)  [unwired: 1 in]
        n81 = Equal To 0?(x=w420) -> (x = 0?=w417:bool)
        n82 = Not Equal To 0?(x=w419) -> (x != 0?=w418:bool)
        n83 = And(x=w417, y=w418) -> (x .and. y?=w411:bool)
        n84 = call "setnag_o2_gauge_subVI.vi"("setnag info in"=w390) -> ("Cluster"=→"Waveform Chart":cluster{"Numeric Control":dbl}, "Numeric Control out"=w452:dbl, "Array"=→"O2 sensor output":dbl[], "String"=w336:string)  [unwired: 7 in]
        n85 = Unbundle(w398) -> ("Numeric Control"=→"O2 Concentration (PPM)":dbl, "Cluster"=→"Waveform Chart 6":cluster{"Numeric Control":dbl}, "String"=w373:string, "error out"=w395:errorcluster)
        n86 = And(x=w350, y=w411) -> (x .and. y?=w387:bool)
        n87 = Greater?(x=w308, y=w321) -> (0:w320:bool)
        n88 = Less?(x=w309, y=w321) -> (x < y?=w319:bool)
        n89 = Or(x=w387, y="Stop") -> (x .or. y?=w412:bool)
        n90 = Bundle("String"=w336, "String"=w373) -> (w372:cluster{"String":string, "String":string})  [unwired: 1 in]
        n91 = call "Arduino read multiple frequencies cristains filter.vi"("main loop iteration number"=w325, "arduino addresses in"=w330, "arduinos on?"=w327) -> ("arduino addresses out"=w328:T25, "arduino frequencies out"=w329:T26, "arduinos on"=w326:bool)  [unwired: 6 in]
        n92 = Less?(x=w308, y=w311) -> (x < y?=w305:bool)
        n93 = Greater?(x=w309, y=w311) -> (0:w306:bool)
        n94 = Decrement(x=w302) -> (x-1=w301:i32)
        n95 = Unbundle("Pressure parameters cluster") -> ("valve % open"=w362:dbl, "Desired pressure"=w364:dbl, "Vapor sccm"=w365:sgl, "Gas sccm"=w366:sgl, "Valve mode"=w367:enum32{"% Open", "Torr "}, "Pressure Mode"=w368:enum32{"Abs. pressure", " Part. pressure"}, "analyte partial pressure"=w369:dbl, "Turbo pump\nauto on"=w310:bool, "read pressure"=w322:dbl)  [unwired: 3 out]
        n96 = Compound Arithmetic op=AND(w310, w307, w319, w320) -> (w316:bool)
        n97 = Compound Arithmetic op=AND(w310, w307, w306, w305) -> (w304:bool)
        n98 = Bundle("valve % open"=w362, "Desired pressure"=w364, "Vapor sccm"=w365, "Gas sccm"=w366, "Valve mode"=w367, "Pressure Mode"=w368, "analyte partial pressure"=w369) -> (w361:T27)  [unwired: 1 in]
        n99 = Index Array(array=w300, index (row)=w301, index (col)=4 ("disabled index (col)")) -> (element=w288:string)
        n100 = call "plot_usr_seq_selectableDisplay.vi"("Display"=w298, "User-defined sequence"=w300) -> ("Sequence Preview"=w299:cluster{dbl[], dbl[]}[])  [unwired: 9 in]
        n101 = property on="Sequence\npreview" class="XYGraph (strict)"("Value"=w299) -> ()  [unwired: 2 in, 2 out]
        n102 = call "Elapsed Time"() -> ("Present (s)"=w357:dbl, "Elapsed Time (s)"=w401:dbl)  [unwired: 12 in, 6 out]
        n103 = Bundle("User-defined\nsequence"=w300, "Present (s)"=w357, "current  step # in"=w349, "sequence end time in"=w353) -> (w358:T28)  [unwired: 1 in]
        n104 = call "Pressure_control_subVI _newturbo.vi"("Run Sequence"=w286, "user sequence, present (s) in, current step in, seq time in"=w358, "pressure parameters in"=w361, "pressure control on?/daq IDs/errors"=w323) -> ("current step # out, shift register time out, seq button on?"=w356:T29, "sequence over? USE THIS TO REINITIALIZE RUN SEQUENCE BUTTON SO PROGRAM ENDS"=w346:bool, "save press/RH/gasflow/vaporflow - read valve position/pressure/vaporflow/gasflow"=w345:T30, "pressure control on?/daq IDs/errors out"=w347:T31, "sequence end date/time string"=w348:string, "pressure_setpoint"=w332:string)  [unwired: 2 in]
        n105 = case shown="True" w316 {
          tunnel: w318 -> [w500 w503]
          tunnel: w317 -> [w499 w504]
          tunnel: [w500 w502] -> w315
          tunnel: [w499 w501] -> w314
          frame False {
          }
          frame True {
            n106 = Concatenate Strings("#000TMPON" ("write buffer 2"), "\r", "\n") -> (w505:string)
            n107 = VISA Write(VISA resource name=w503, write buffer=w505, error in (no error)=w504) -> (VISA resource name out=w502:refnum<visa-resource-name>, error out=w501:errorcluster)  [unwired: 1 out]
          }
        }
        n108 = call "Elapsed Time2"("Set Start Time (s)"=w357) -> ("Elapsed Time (s)"=w385:dbl)  [unwired: 11 in, 7 out]
        n109 = case shown="True" w346 {
          frame False {
          }
          frame True {
            n110 = property on="Run Sequence" class="Bool (strict)"("Value"=FALSE ("Run Sequence")) -> ()  [unwired: 2 in, 2 out]
          }
        }
        n111 = Unbundle(w345) -> ("press/RH/gas/vapor"=w344:T32, "Cluster"=w343:T33)
        n112 = property on="Sequence end time" class="Str"("Value"=w348) -> ()  [unwired: 2 in, 2 out]
        n113 = event shown="[1] \"Clear all charts\": Value Change" {
          selector: _ -> [_ _ _ _ _]
          dyn-events: _ -> [_ _ _ _ _]
          timeout: 50 -> [_ _ _ _ _]
          tunnel: w300 -> [_ _ _ w538 _]
          tunnel: w385 -> [_ _ _ _ _]
          tunnel: w384 -> [w531 _ _ _ _]
          tunnel: [w531 _ _ _ _] -> w383
          event Timeout {
            n114 = event-data() -> ()  [unwired: 1 in, 1 out]
          }
          event "Clear all charts": Value Change {
            (unwired) T34 [] ("History Data")
            w535 = cluster{dbl}[] [] ("History Data")
            w536 = cluster{"Resistance":sgl}[] [] ("History Data")
            w534 = dbl[] [] ("History Data")
            (unwired) cluster{dbl, "Resistance out":dbl}[] [] ("History Data")
            n115 = event-data() -> ()  [unwired: 1 in, 1 out]
            n116 = property on="K-6430" class="WFChart (strict)"("History Data"=w536) -> ()  [unwired: 2 in, 2 out]
            n117 = property on="arduino qcm 1" class="WFChart (strict)"("History Data"=w534) -> ()  [unwired: 2 in, 2 out]
            n118 = property on="Waveform Chart" class="WFChart (strict)"("History Data"=w535) -> ()  [unwired: 2 in, 2 out]
            n119 = property on="QCM plot" class="WFChart (strict)"("History Data"=T13 []) -> ()  [unwired: 2 in, 2 out]
            n120 = property on="arduino qcm 6" class="WFChart (strict)"("History Data"=w534) -> ()  [unwired: 2 in, 2 out]
            n121 = property on="K-2100 (Ohm)" class="WFChart (strict)"("History Data"=w536) -> ()  [unwired: 2 in, 2 out]
            n122 = property on="arduino qcm stack plot" class="WFChart (strict)"("History Data"=T12 []) -> ()  [unwired: 2 in, 2 out]
            n123 = property on="arduino qcm 3" class="WFChart (strict)"("History Data"=w534) -> ()  [unwired: 2 in, 2 out]
            n124 = property on="arduino qcm 2" class="WFChart (strict)"("History Data"=w534) -> ()  [unwired: 2 in, 2 out]
            n125 = property on="pressure chart" class="WFChart (strict)"("History Data"=w535) -> ()  [unwired: 2 in, 2 out]
            n126 = property on="arduino qcm 4" class="WFChart (strict)"("History Data"=w534) -> ()  [unwired: 2 in, 2 out]
            n127 = property on="arduino qcm 5" class="WFChart (strict)"("History Data"=w534) -> ()  [unwired: 2 in, 2 out]
          }
          event "Sequence cluster.Clear sequence": Value Change {
            n128 = event-data() -> ()  [unwired: 1 in, 1 out]
            n129 = property on="User-defined\nsequence" class="Tbl (strict)"("Value"=string[][] []) -> ()  [unwired: 2 in, 2 out]
          }
          event "Sequence cluster.Save sequence": Value Change {
            n130 = event-data() -> ()  [unwired: 1 in, 1 out]
            n131 = call-poly <vilib>:"Write To Spreadsheet File.vi"("2D data"=w538) -> ()  [unwired: 7 in, 1 out]
          }
          event "Sequence cluster.Import sequence file": Value Change {
            n132 = event-data() -> ()  [unwired: 1 in, 1 out]
            n133 = call-poly <vilib>:"Read From Spreadsheet File.vi"() -> ("all rows"=w539:string[][])  [unwired: 7 in, 4 out]
            n134 = property on="User-defined\nsequence" class="Tbl (strict)"("Value"=w539) -> ()  [unwired: 2 in, 2 out]
          }
        }
        n135 = Fract/Exp String To Number(string=w288) -> (number=w287:dbl)  [unwired: 3 in, 1 out]
        n136 = Select(t=w287, s=w286, f="Applied Voltage (V)") -> (s? t:f=w290:dbl)
        n137 = case shown="True" w291 {
          selector: w291 -> [w458 w464]
          tunnel: ["" w463] -> w284
          tunnel: [w455 w462] -> w285
          tunnel: w293 -> [w457 w461]
          tunnel: w292 -> [w456 w460]
          tunnel: w290 -> [_ w459]
          frame False {
            n138 = Bundle(w458, "VISA resource name out"=w457, "error out"=w456) -> (w455:T18)  [unwired: 1 in]
          }
          frame True {
            n139 = case shown="\"K-2420 Apply bias\"" "K-2420 tab control" {
              tunnel: w461 -> [w470 w482]
              tunnel: w460 -> [w469 w481]
              tunnel: [w468 w479] -> w462
              tunnel: w464 -> [w467 w480]
              tunnel: [w466 w478] -> w463
              tunnel: w459 -> [_ w477]
              frame "K-2420 Measure", Default {
                w471 = i16 15 ("width (-)")
                n140 = call-poly "Read.vi"("VISA resource name"=w470, "error in (no error)"=w469) -> ("VISA resource name out"=w474:refnum<visa-resource-name>, "Resistance"=w472:sgl, "error out"=w473:errorcluster)  [unwired: 7 in, 4 out]
                n141 = Bundle("Resistance"=w472) -> (→"K-2420 2":cluster{"Resistance":sgl})  [unwired: 1 in]
                n142 = Number To Engineering String(2:w471, 3:w471, 4:w472) -> (0:w466:string)  [unwired: 1 in]
                n143 = Bundle(w467, "VISA resource name out"=w474, "error out"=w473) -> (w468:T18)  [unwired: 1 in]
              }
              frame "K-2420 Apply bias" {
                w485 = u16 0 items=["Voltage", "Current"] ("Source Mode  (0: Voltage)")
                w486 = i16 15 ("width (-)")
                n144 = call "Configure Output.vi"("Source Mode  (0: Voltage)"=w485, "error in (no error)"=w481, "Output Level (0)"=w477, "VISA resource name"=w482) -> ("error out"=w483:errorcluster, "VISA resource name out"=w484:refnum<visa-resource-name>)  [unwired: 6 in]
                n145 = call-poly "Read.vi"("VISA resource name"=w484, "error in (no error)"=w483) -> ("VISA resource name out"=w488:refnum<visa-resource-name>, "error out"=w487:errorcluster)  [unwired: 7 in, 5 out]
                n146 = Bundle("Applied Voltage (V)"=w477) -> (→"K-2420 4":cluster{"Applied Voltage (V)":dbl})  [unwired: 1 in]
                n147 = Number To Engineering String(2:w486, 3:w486, 4:w477) -> (0:w478:string)  [unwired: 1 in]
                n148 = Bundle(w480, "VISA resource name out"=w488, "error out"=w487) -> (w479:T18)  [unwired: 1 in]
              }
            }
          }
        }
        n149 = Fract/Exp String To Number(string=w329) -> (number=w324:T1)  [unwired: 3 in, 1 out]
        n150 = Unbundle(w343) -> ("Valve position (%)"=w342:dbl, "read pressure"=w337:dbl, "read vapor flow"=w341:dbl, "read gas flow"=w340:dbl)
        n151 = Unbundle("Data logging settings") -> ("Save during sequence only"=w414:bool, "Save now"=w416:bool, "sec between data points"=w403:dbl, "Save sample names"=w297:T35, "Experiment Notes"=w295:string, "Cluster"=w294:cluster{"Gas:":string, "Vapor:":string})  [unwired: 1 out]
        n152 = property on="Valve position (%)" class="DigNum (strict)"("Value"=w342) -> ()  [unwired: 2 in, 2 out]
        n153 = case shown="True" w326 {
          tunnel: w324 -> [_ w510]
          frame False {
          }
          frame True {
            n154 = Unbundle(w510) -> ("mean"=w512:dbl, "mean"=w511:dbl, "mean"=w517:dbl, "mean"=w516:dbl, "mean"=w515:dbl, "mean"=w514:dbl)
            n155 = Bundle("mean"=w512, "mean"=w512, "mean"=w511, "mean"=w511, "mean"=w517, "mean"=w517, "mean"=w516, "mean"=w516, "mean"=w515, "mean"=w515, "mean"=w514, "mean"=w514) -> (→"ArduinoQCM cluster":T36)  [unwired: 1 in]
            "arduino qcm stack plot" <- w510
          }
        }
        n156 = And(x=w286, y=w414) -> (x .and. y?=w413:bool)
        n157 = Subtract(x=w401, y=w383) -> (x-y=w400:dbl)
        n158 = Bundle("read pressure"=w337) -> (→"pressure chart":cluster{"read pressure":dbl})  [unwired: 1 in]
        n159 = property on="read pressure" class="DigNum (strict)"("Value"=w337) -> ()  [unwired: 2 in, 2 out]
        n160 = Or(x=w413, y=w416) -> (x .or. y?=w410:bool)
        "saving data?" <- w410
        n161 = case shown="True" w304 {
          tunnel: w315 -> [w490 w493]
          tunnel: w314 -> [w489 w494]
          tunnel: [w490 w492] -> w312
          tunnel: [w489 w491] -> w313
          frame False {
          }
          frame True {
            n162 = Concatenate Strings("#000TMPOFF" ("write buffer 2"), "\r", "\n") -> (w495:string)
            n163 = VISA Write(VISA resource name=w493, write buffer=w495, error in (no error)=w494) -> (VISA resource name out=w492:refnum<visa-resource-name>, error out=w491:errorcluster)  [unwired: 1 out]
          }
        }
        n164 = Divide(x=w400, y=60.0) -> (x/y=w375:dbl)
        "Elapsed time (min)" <- w375
        n165 = property on="read vapor flow" class="DigNum (strict)"("Value"=w341) -> ()  [unwired: 2 in, 2 out]
        n166 = Multiply(x=w403, y=u32 1000 ("x")) -> (x*y=w435:dbl)
        n167 = Bundle("String data out"=w382, w394, w284, w393) -> (w388:T37)  [unwired: 1 in]
        n168 = Wait (ms)(milliseconds to wait=w435) -> ()  [unwired: 1 out]
        n169 = property on="read gas flow" class="DigNum (strict)"("Value"=w340) -> ()  [unwired: 2 in, 2 out]
        n170 = call "data_headers_subVI_w_gases.vi"("gas/vapor names"=w294, "Experiment Notes"=w295, "Sample names"=w297) -> ("data headers"=w296:string[])  [unwired: 8 in]
        n171 = Get Date/Time In Seconds() -> (seconds since 1Jan1904=w453:timestamp)
        n172 = Number To Engineering String ("elapsed time (min)")(4:w375) -> (0:w380:string)  [unwired: 3 in]
        n173 = Unbundle(w356) -> ("current  step # in"=w335:i32, "sequence end time in"=w355:timestamp, "Boolean"=w354:bool)
        n174 = Format Date/Time String(time format string (%c)="%Y-%m-%d %H:%M:%S%2u", seconds (now)=w453) -> (date/time string=w432:string)  [unwired: 1 in]
        n175 = Unbundle(w388) -> ("String data out"=w379:string, w378:string, w377:string, w376:string)
        n176 = Unbundle(w431) -> ("String"=w381:string, "String"=w434:string, "String"=w433:string)
        n177 = Unbundle(w372) -> ("String"=w371:string, "String"=w370:string)
        n178 = Unbundle(w344) -> ("pressure"=w426:string, "RH"=w425:string, "gas flow"=w424:string, "vapor flow"=w423:string)
        n179 = Unbundle ("arduino 1-6")(w329) -> ("mean"=w333:string, "mean"=w430:string, "mean"=w429:string, "mean"=w428:string, "mean"=w427:string, "mean"=w331:string)
        n180 = Increment(x=w335) -> (x+1=w334:i32)
        n181 = Build Array(w432, w380, w379, w378, w377, w376, w381, w434, w433, w371, w370, w426, w425, w424, w423, w332, w333, w430, w429, w428, w427, w331) -> (w440:string[])
        n182 = property on="Current\nstep" class="DigNum (strict)"("Value"=w334) -> ()  [unwired: 2 in, 2 out]
        "State date/time" <- w374
      }
      n183 = Unbundle(w88) -> (w87:bool, "VISA resource name out"=w86:refnum<visa-resource-name>, "error out"=w85:errorcluster)
      n184 = Unbundle(w84) -> ("Boolean"=w83:bool, "VISA out"=w82:refnum<visa-resource-name>, "error out"=w81:errorcluster)
      n185 = call-poly <vilib>:"Write To Spreadsheet File.vi"("1D data"=w52, "file path (dialog if empty)"=w69) -> ("new file path (Not A Path if cancelled)"=w73:path)  [unwired: 6 in]
      n186 = Unbundle(w62) -> (w67:bool, "VISA resource name out"=w66:refnum<visa-resource-name>, "error out"=w65:errorcluster)
      n187 = Unbundle(w34) -> ("Boolean"=w33:bool, "task out"=w16:refnum<k21>, "error out"=w15:errorcluster, "task out"=w14:refnum<k21>, "error out"=w13:errorcluster, "VISA resource name out"=w12:refnum<visa-resource-name>, "error out"=w11:errorcluster)
      n188 = call "arduino_close_subIV.vi"("arduino 1-6 addresses and errors out"=w54, "arduinos on?"=w53) -> ()  [unwired: 10 in]
      n189 = case shown="True" w46 {
        tunnel: w45 -> [_ w108]
        tunnel: w44 -> [w105 w107]
        tunnel: [w105 w106] -> w43
        frame False {
        }
        frame True {
          n190 = call "Close.vi"("VISA resource name"=w108, "error in (no error)"=w107) -> ("error out"=w106:errorcluster)  [unwired: 17 in]
        }
      }
      n191 = flat-sequence {
        tunnel: w21 -> [w104]
        tunnel: [w104] -> w20
        frame #0 {
          n192 = property on="saving data?" class="Bool (strict)"("Value"=FALSE ("saving data?")) -> ()  [unwired: 2 in, 2 out]
        }
      }
      n193 = Unbundle(w79) -> ("Boolean"=w78:bool, "VISA resource name out"=w77:refnum<visa-resource-name>, "error out"=w76:errorcluster)
      n194 = case shown="True" w33 {
        tunnel: [errorcluster {"status"=FALSE, "code"=0, "source"=""} ("error out") w133] -> w38
        tunnel: w16 -> [_ w132]
        tunnel: w15 -> [_ w131]
        tunnel: w14 -> [_ w130]
        tunnel: w13 -> [_ w127]
        tunnel: w12 -> [_ w128]
        tunnel: w11 -> [_ w129]
        tunnel: w7 -> [_ w124]
        tunnel: w6 -> [_ w123]
        frame False {
        }
        frame True {
          n195 = call <vilib>:"DAQmx Stop Task.vi"("task/channels in"=w132, "error in"=w131) -> ("task out"=w139:refnum<k21>, "error out"=w138:errorcluster)  [unwired: 12 in]
          n196 = call <vilib>:"DAQmx Stop Task.vi"("task/channels in"=w130, "error in"=w127) -> ("task out"=w140:refnum<k21>, "error out"=w141:errorcluster)  [unwired: 12 in]
          n197 = VISA Clear(VISA resource name=w128, error in (no error)=w129) -> (VISA resource name out=w137:refnum<visa-resource-name>, error out=w136:errorcluster)
          n198 = VISA Close(VISA resource name=w124, error in (no error)=w123) -> (error out=w125:errorcluster)
          n199 = VISA Close(VISA resource name=w137, error in (no error)=w136) -> (error out=w126:errorcluster)
          n200 = call <vilib>:"DAQmx Clear Task.vi"("task in"=w139, "error in"=w138) -> ("error out"=w135:errorcluster)  [unwired: 13 in]
          n201 = call <vilib>:"DAQmx Clear Task.vi"("task in"=w140, "error in"=w141) -> ("error out"=w134:errorcluster)  [unwired: 13 in]
          n202 = Merge Errors(w135, w134, w126, w125) -> (w133:errorcluster)
        }
      }
      n203 = case shown="True" w87 {
        tunnel: w86 -> [_ w257]
        tunnel: w85 -> [w254 w256]
        tunnel: [w254 w255] -> w89
        frame False {
        }
        frame True {
          n204 = call "Enable Output.vi"("error in (no error)"=w256, "Enable Output (T: Enable)"=FALSE, "VISA resource name"=w257) -> ("error out"=w258:errorcluster, "VISA resource name out"=w260:refnum<visa-resource-name>)  [unwired: 7 in]
          n205 = call "Close.vi"("error in (no error)"=w258, "VISA resource name"=w260) -> ("error out"=w255:errorcluster)  [unwired: 9 in]
        }
      }
      n206 = case shown="True" w67 {
        tunnel: w66 -> [_ w172]
        tunnel: w65 -> [w170 w171]
        tunnel: [w170 w173] -> w61
        frame False {
        }
        frame True {
          n207 = call "Enable Output.vi"("error in (no error)"=w171, "Enable Output (F:Off)"=FALSE ("Output (F:Off)"), "VISA resource name"=w172) -> ("error out"=w174:errorcluster, "VISA resource name out"=w175:refnum<visa-resource-name>)  [unwired: 7 out]
          n208 = call "Close.vi"("error in (no error)"=w174, "VISA resource name"=w175) -> ("error out"=w173:errorcluster)  [unwired: 9 out]
        }
      }
      n209 = case shown="True" w83 {
        tunnel: w81 -> [w240 w243]
        tunnel: [w240 w242] -> w90
        tunnel: w82 -> [_ w241]
        frame False {
        }
        frame True {
          n210 = call "srsQcm200Close.vi"("error in"=w243, "Visa in"=w241) -> ("error out"=w242:errorcluster)  [unwired: 3 in]
        }
      }
      n211 = call-poly <vilib>:"Write To Spreadsheet File.vi"("append to file? (new file:F)"=TRUE, "2D data"=w56, "file path (dialog if empty)"=w73) -> ()  [unwired: 5 in, 1 out]
      n212 = case shown="True" w78 {
        tunnel: w77 -> [_ w210]
        tunnel: w76 -> [w207 w209]
        tunnel: [w207 w208] -> w75
        frame False {
        }
        frame True {
          n213 = VISA Close(VISA resource name=w210, error in (no error)=w209) -> (error out=w208:errorcluster)
        }
      }
      n214 = Merge Errors(w61, w75, w89, w43, w90, w20) -> (w96:errorcluster)
      n215 = call <vilib>:"Simple Error Handler.vi"("error in (no error)"=w38) -> ()  [unwired: 4 in, 5 out]
      n216 = call <vilib>:"Simple Error Handler.vi"("error in (no error)"=w96) -> ()  [unwired: 4 in, 5 out]
    }
  }
